vi "LightFieldChangeBackground.vi"(8 "error in":errorcluster, 10 "FilePath":string, 11 "LightField Automation in":refnum<class "LightField Automation.lvclass">) -> (0 "error out":errorcluster, 3 "LightField Automation out":refnum<class "LightField Automation.lvclass">)   [LabVIEW 2018]
uses:
  <userlib>/LightField Add-in and Automation SDK/Samples/LabVIEW Automation/lightfield-automation-labview/LightField Automation.lvclass
  C:/Program Files/Princeton Instruments/LightField/PrincetonInstruments.LightFieldAddInSupportServices.dll
  Program Files/Princeton Instruments/LightField/PrincetonInstruments.LightFieldAddInSupportServices.dll
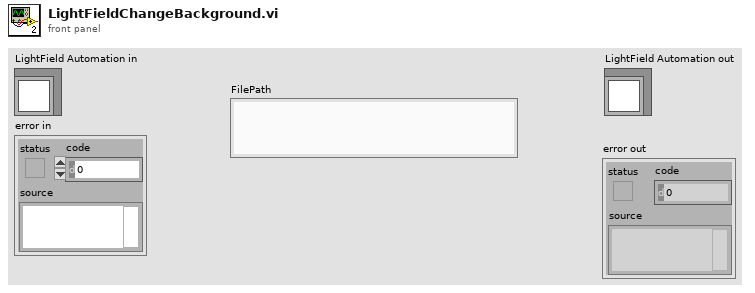
[diagram p1: front panel]
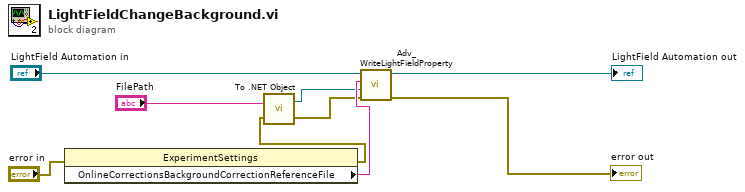
[diagram p0: block diagram]
diagram:
  n1 = property class="ExperimentSettings"(error in="error in") -> (error out=w4:errorcluster, "OnlineCorrectionsBackgroundCorrectionReferenceFile"=w5:string)  [unwired: 1 in, 1 out]
  n2 = call <vilib>:"To .NET Object.vi"("error in (no error)"=w4, "anything"="FilePath") -> ("error out"=w2:errorcluster, ".NET object"=w3:refnum<k24>)
  n3 = call <userlib>:"Adv_WriteLightFieldProperty.vi"("error in (no error)"=w2, "value"=w3, "setting"=w5, "LightField Automation in"="LightField Automation in") -> ("error out"=→"error out":errorcluster, "LightField Automation out"=→"LightField Automation out":refnum<class "LightField Automation.lvclass">)  [unwired: 6 in]
